vi "PathToQuotedString.vi"(4 "Path":path) -> (1 "String":string)   [LabVIEW 2022 SP3]
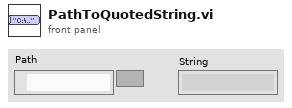
[diagram p1: front panel]
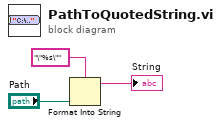
[diagram p0: block diagram]
diagram:
  n1 = Format Into String(format string="\"%s\"" ("string"), "Path") -> (resulting string=→"String":string)  [unwired: 2 in, 1 out]
